vi "process.vi"(8 "error in":errorcluster, 9 "result allocation":T1, 10 "parameters":T1, 11 "module in":refnum<class "TEST RUNTIME.lvclass">) -> (0 "error out":errorcluster, 1 "results":T1, 2 "parameter allocation":T1, 3 "module out":refnum<class "TEST RUNTIME.lvclass">)   [LabVIEW 2013, in "configuration tests.lvlib" / "TEST RUNTIME.lvclass"]
doc: "Provides an interface for information processing by a module at runtime. While this interface performs no operations, a child should provide an override which may process data in any manner necessary."
uses:
  TEST RUNTIME.lvclass
  <vilib>/NI/Tag Bus/table/data table.ctl
  TEST RUNTIME.lvclass/TEST RUNTIME.ctl
  <vilib>/NI/Tag Bus/table/data table.lvlib
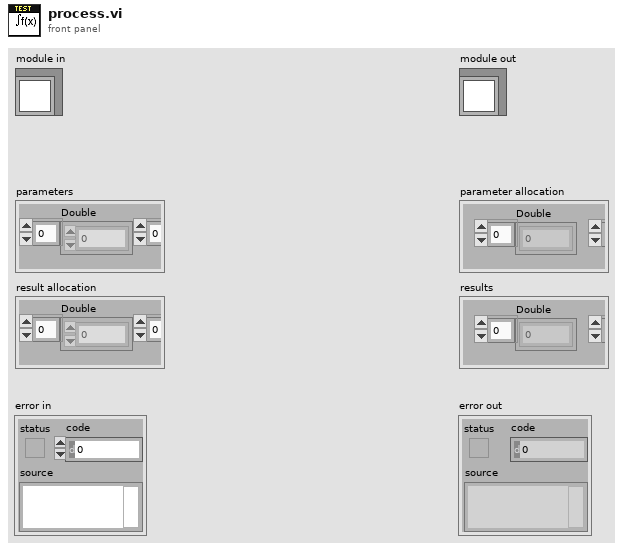
[diagram p1: front panel]
types:
  T1 = typedef "tag bus.lvlib/data table.lvlib/data table.ctl" = cluster{"Double":dbl[], "Single":sgl[], "I64":i64[], "I32":i32[], "I16":i16[], "I8":i8[], "U64":u64[], "U32":u32[], "U16":u16[], "U8":u8[], "Boolean":bool[], "String":string[], "Array of Double":cluster{"DBL Array":dbl[]}[], "Array of Single":cluster{"SGL Array":sgl[]}[], "Array of I64":cluster{"I64 Array":i64[]}[], "Array of I32":cluster{"I32 Array":i32[]}[], "Array of I16":cluster{"I16 Array":i16[]}[], "Array of I8":cluster{"I8 Array":i8[]}[], "Array of U64":cluster{"U64 Array":u64[]}[], "Array of U32":cluster{"U32 Array":u32[]}[], "Array of U16":cluster{"U16 Array":u16[]}[], "Array of U8":cluster{"U8 Array":u8[]}[], "Array of Boolean":cluster{"Boolean Array":bool[]}[], "Array of String":cluster{"String Array":string[]}[]}
  T2 = typedef "configuration tests.lvlib/TEST RUNTIME.lvclass/state control.ctl" = cluster{"state":u8, "control index (dbl)":i32, "output index (dbl)":i32}
  T3 = typedef "configuration tests.lvlib/TEST RUNTIME.lvclass/control module.ctl" = cluster{"setpoint index (dbl)":i32, "proc var index (dbl)":i32, "output index (dbl)":i32, "output range":cluster{"output high":dbl, "output low":dbl}, "Kp":dbl, "Ki":dbl, "Kd":dbl, "error int":dbl, "last error":dbl}
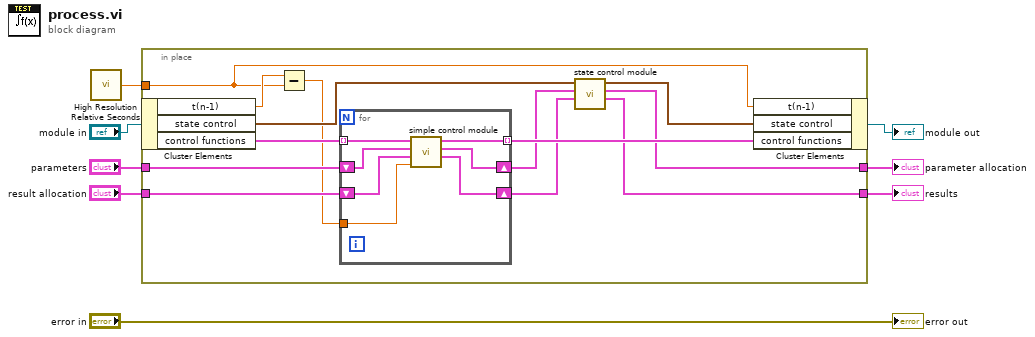
[diagram p0: block diagram]
diagram:
  n1 = call <vilib>:"High Resolution Relative Seconds.vi"() -> ("relative seconds"=w1:dbl)
  n2 = in-place {
    in-place-border: "parameters" -> [w21]
    in-place-border: "result allocation" -> [w20]
    in-place-border: [w13] -> w3
    in-place-border: [w15] -> w2
    in-place-border: w1 -> [w9]
    n3 = in-place-cluster #1("module in") -> ("t(n-1)"=w11:dbl, "state control"=w17:T2, "control functions"=w19:T3[])
    n4 = Subtract(x=w11, y=w9) -> (x-y=w10:dbl)
    n5 = for {
      tunnel: w10 -> [w22]
      shift-right: [w26] -> w16
      shift-left: w21 -> [w25]
      shift-right: [w23] -> w12
      shift-left: w20 -> [w24]
      tunnel: w19 -> [w28] mode=indexing
      tunnel: [w27] -> w18 mode=indexing
      n6 = call "simple control module.vi"("dt"=w22, "results in"=w24, "parameters in"=w25, "sample control module"=w28) -> ("results out"=w23:T1, "parameters out"=w26:T1, "sample control module out"=w27:T3)  [unwired: 5 in]
    }
    n7 = call "state control module.vi"("results in"=w12, "parameters in"=w16, "state control in"=w17) -> ("results out"=w13:T1, "parameters out"=w15:T1, "state control out"=w14:T2)  [unwired: 6 in]
    n8 = in-place-cluster #1("t(n-1)"=w9, "state control"=w14, "control functions"=w18) -> (→"module out":refnum<class "TEST RUNTIME.lvclass">)
  }
  "results" <- w3
  "parameter allocation" <- w2
  "error out" <- "error in"
